vi "DeviceSetNiAuthPasswordRequest_Create.vi"(7 "Header":T2, 8 "error in (no error)":errorcluster, 9 "DeviceSetNiAuthPasswordRequest":T1, 10 "SendTo":string, 11 "ReplyTo":string) -> (0 "error out":errorcluster, 3 "Message":T4)   [LabVIEW 2017]
uses:
  <vilib>/addons/InsightCM/MessageBus/Base/controls/Message.ctl
  <vilib>/addons/InsightCM/MessageBus/Base/controls/MessageHeader.ctl
  <vilib>/addons/InsightCM/MessageBus/Base/controls/KeyValuePair.ctl
  <vilib>/addons/InsightCM/MessageBus/MessageLibrary/Device/controls/DeviceSetNiAuthPasswordRequestBody.ctl
  <vilib>/addons/InsightCM/MessageBus/Base/controls/MessageClassType.ctl
  <vilib>/addons/InsightCM/Utilities/PropertyHelpers/PropertyHelpers.lvlib
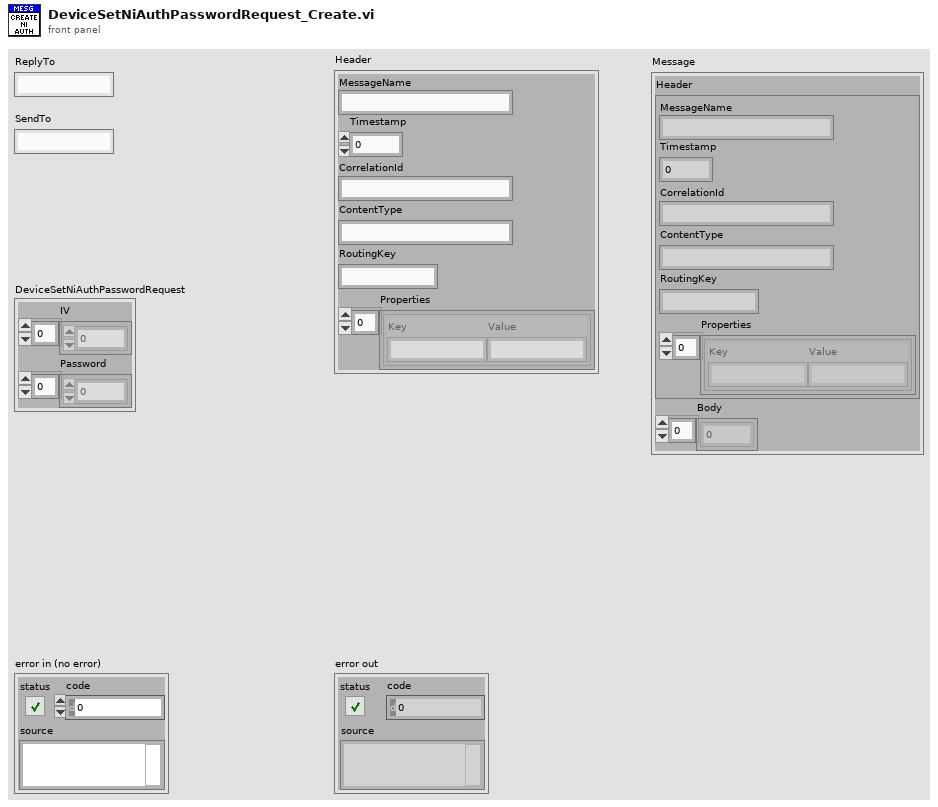
[diagram p1: front panel]
types:
  T1 = typedef "DeviceSetNiAuthPasswordRequestBody.ctl" = cluster{"IV":u8[], "Password":u8[]}
  T2 = typedef "MessageHeader.ctl" = cluster{"MessageName":string, "Timestamp":i64, "CorrelationId":string, "ContentType":string, "RoutingKey":string, "Properties":T3[]}
  T3 = typedef "KeyValuePair.ctl" = cluster{"Key":string, "Value":string}
  T4 = typedef "Message.ctl" = cluster{"Header":T2, "Body":u8[]}
  T5 = typedef "MessageClassType.ctl" = enum16{"Request", "Response", "Broadcast", "RoutedMessage"}
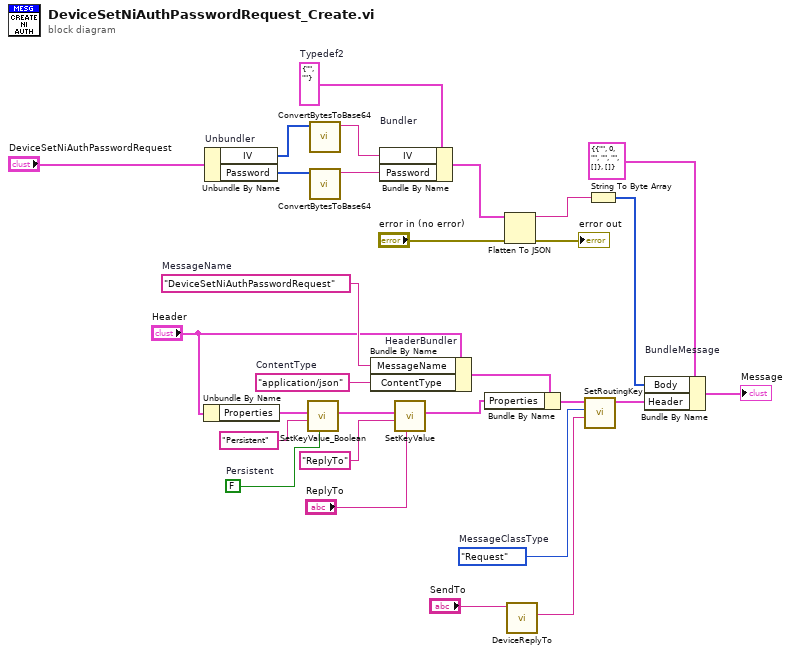
[diagram p0: block diagram]
diagram:
  w5 = cluster{"IV":string, "Password":string} {"IV"="", "Password"=""}  # Typedef2
  w25 = MessageClassType."Request"  # MessageClassType
  w20 = FALSE  # Persistent
  w26 = "DeviceSetNiAuthPasswordRequest"  # MessageName
  w23 = "application/json"  # ContentType
  n1 = Unbundle By Name("Header") -> ("Properties"=w22:T3[])
  n2 = Unbundle By Name "Unbundler"("DeviceSetNiAuthPasswordRequest") -> ("IV"=w4:u8[], "Password"=w2:u8[])
  n3 = call <vilib>:"SetKeyValue_Boolean.vi"("value"=w20, "key"="Persistent" ("Key"), "key value pairs"=w22) -> ("key value pairs out"=w18:T3[])  [unwired: 8 in]
  n4 = call <vilib>:"ConvertBytesToBase64.vi"("U8 array"=w4) -> ("base64 encoded"=w3:string)  [unwired: 10 in]
  n5 = call <vilib>:"ConvertBytesToBase64.vi"("U8 array"=w2) -> ("base64 encoded"=w1:string)  [unwired: 10 in]
  n6 = Bundle By Name "HeaderBundler"(cluster="Header", "MessageName"=w26, "ContentType"=w23) -> (w16:T2)
  n7 = Bundle By Name "Bundler"(cluster=w5, "IV"=w3, "Password"=w1) -> (w6:cluster{"IV":string, "Password":string})
  n8 = call <vilib>:"SetKeyValue.vi"("value"="ReplyTo", "key"="ReplyTo" ("Key"), "key value pairs"=w18) -> ("key value pairs out"=w15:T3[])  [unwired: 8 in]
  n9 = Bundle By Name(cluster=w16, "Properties"=w15) -> (w17:T2)
  n10 = Flatten To JSON(anything=w6, error in (no error)="error in (no error)") -> (JSON string=w8:string, 11:→"error out":errorcluster)  [unwired: 1 in]
  n11 = call <vilib>:"DeviceReplyTo.vi"("Device"="SendTo") -> ("ReplyTo"=w9:string)  [unwired: 10 in]
  n12 = call <vilib>:"SetRoutingKey.vi"("SendTo"=w9, "MessageClassType"=w25, "Message Header in"=w17) -> ("Message Header out"=w19:T2)  [unwired: 8 in]
  n13 = String To Byte Array(string=w8) -> (unsigned byte array=w28:u8[])
  n14 = Bundle By Name "BundleMessage"(cluster=T4 {"Header"={"MessageName"="", "Timestamp"=0, "CorrelationId"="", "ContentType"="", "RoutingKey"="", "Properties"=[]}, "Body"=[]} ("Message"), "Body"=w28, "Header"=w19) -> (→"Message":T4)
